vi "2D Array to Dynamic Data.vi"(7 "Time Stamp Control":timestamp, 8 "Error In":errorcluster, 10 "Channels":string[](array[string]), 11 "Array":dbl[][](array[numeric])) -> (0 "Error Out":errorcluster, 2 "Channels out":string[](array[string]), 3 "Dynamic Data Type":dynamicdata(graph))   [LabVIEW 2016]
panel:
  out "Array 2":dbl[](array[numeric])
  out "channel number":i32
  out "rows":i32
  in  "file path":path=path "C:/Data/test.tdms"
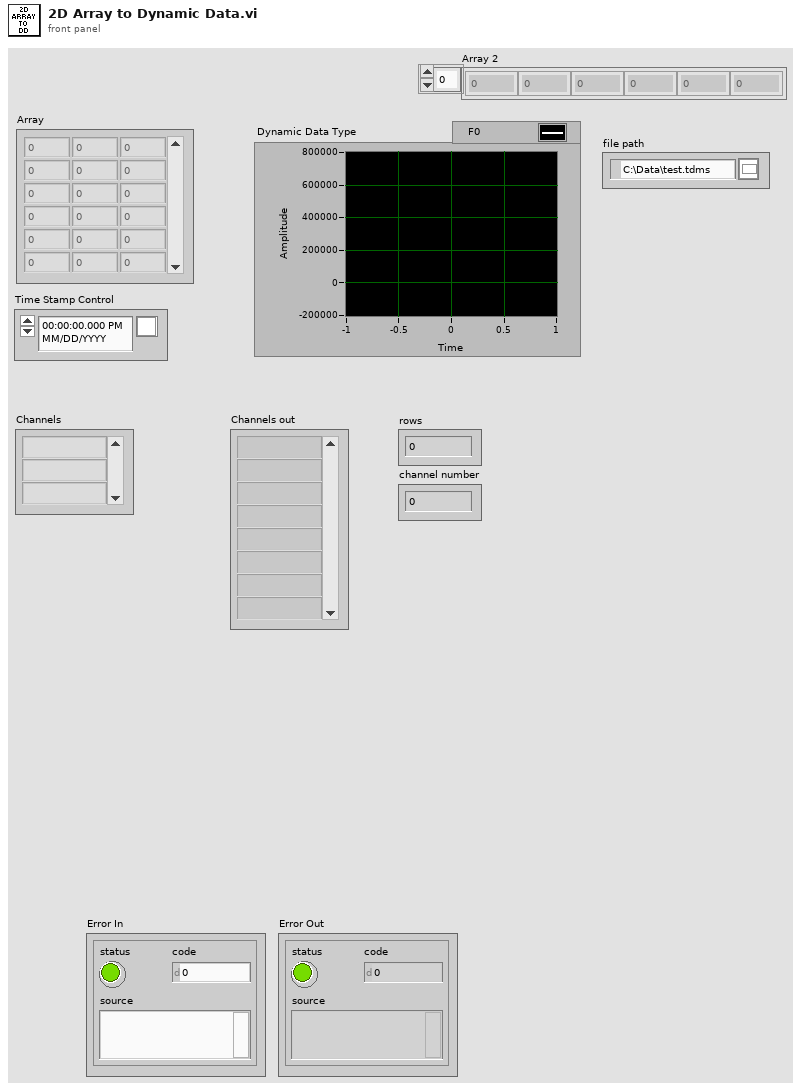
[diagram p1: front panel]
types:
  T1 = enum16{"open", "open or create", "create or replace", "create", "open (read-only)"}
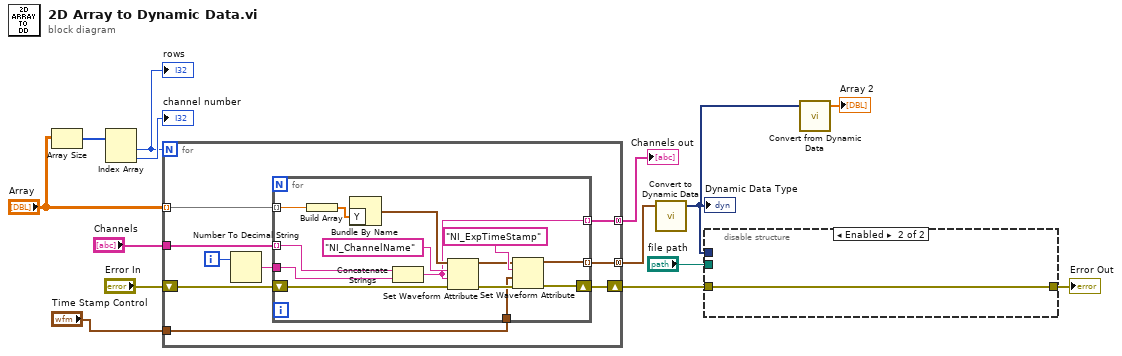
[diagram p0: block diagram]
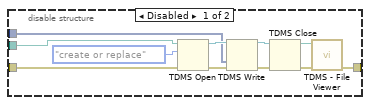
[diagram p2: hidden frame]
diagram:
  n1 = Array Size(array="Array") -> (size(s)=w13:i32[])
  n2 = Index Array(array=w13) -> (element #1=w11:i32, element #2=→"channel number":i32)  [unwired: 2 in]
  "rows" <- w11
  n3 = for {
    N: w11 -> [_]
    tunnel: "Channels" -> [w22]
    tunnel: [w20] -> w10 mode=concatenating
    tunnel: "Array" -> [w19] mode=indexing
    tunnel: [w18] -> w9 mode=concatenating
    shift-right: [w16] -> w8
    shift-left: "Error In" -> [w17]
    tunnel: "Time Stamp Control" -> [w15]
    i -> [w23]
    n4 = Number To Decimal String(number=w23) -> (decimal integer string=w21:string)  [unwired: 1 in]
    n5 = for {
      tunnel: w22 -> [w37] mode=indexing
      tunnel: w21 -> [w36]
      tunnel: [w30] -> w20 mode=indexing
      tunnel: w19 -> [w35] mode=indexing
      tunnel: [w24] -> w18 mode=indexing
      shift-right: [w28] -> w16
      shift-left: w17 -> [w32]
      tunnel: w15 -> [w27]
      n6 = Build Array(w35) -> (w34:dbl[])
      n7 = Bundle By Name("Y"=w34) -> (w33:waveform(dbl))  [unwired: 1 in]
      n8 = Concatenate Strings(w37, w36) -> (w30:string)
      n9 = Set Waveform Attribute(4:w32, 5:w30, 6:"NI_ChannelName" ("name"), 7:w33) -> (0:w29:errorcluster, 3:w25:waveform(dbl))  [unwired: 1 out]
      n10 = Set Waveform Attribute(4:w29, 5:w27, 6:"NI_ExpTimeStamp" ("name"), 7:w25) -> (0:w28:errorcluster, 3:w24:waveform(dbl))  [unwired: 1 out]
    }
  }
  "Channels out" <- w10
  n11 = call "Convert to Dynamic Data"("Array of Waveforms"=w9) -> ("Dynamic Data Type"=w3:dynamicdata)  [unwired: 3 in]
  "Dynamic Data Type" <- w3
  n12 = disable-structure shown="Enabled" {
    disable-tunnel: "file path" -> [w48 _]
    disable-tunnel: w3 -> [w44 _]
    disable-tunnel: w8 -> [w39 w49]
    disable-tunnel: [w38 w49] -> w4
    frame Disabled {
      n13 = TDMS Open(8:w39, 10:T1."create or replace" ("operation (0:open)"), 11:w48) -> (0:w45:errorcluster, 3:w46:refnum<k34>)  [unwired: 4 in]
      n14 = TDMS Write(0:w46, 9:w44, 11:w45) -> (4:w42:refnum<k34>, 15:w43:errorcluster)  [unwired: 3 in, 2 out]
      n15 = TDMS Close(8:w43, 11:w42) -> (0:w40:errorcluster, 3:w41:path)
      n16 = call <vilib>:"TDMS - File Viewer.vi"("error in (no error)"=w40, "file path"=w41) -> ("error out"=w38:errorcluster)  [unwired: 4 in, 1 out]
    }
    frame Enabled {
    }
  }
  "Error Out" <- w4
  n17 = call "Convert from Dynamic Data"("Dynamic Data Type"=w3) -> ("Array"=→"Array 2":dbl[])  [unwired: 3 in]
